vi "Write and Read Multiple Holding Registers.vi"(4 "read count":u16, 6 "read operation starting address":u16, 8 "error in (no error)":errorcluster, 9 "values to write":u16[](array[numeric]), 10 "write operation starting address":u16, 11 "Modbus master in":refnum<class "Network Master.lvclass">) -> (0 "error out":errorcluster, 1 "values read":u16[](array[numeric]), 3 "Modbus master out":refnum<class "Network Master.lvclass">)   [LabVIEW 2021, in "Network Master.lvclass"]
doc: "Writes and reads values to and from contiguous holding registers. This VI performs the write operation before the read operation. The maximum number of holding registers this VI can write is 121. The maximum number of holding registers this VI can read is 125."
uses:
  Network Master.lvclass
  D:/my_projects/projects/Algorithms/Labview/21/Modbus_v121c/Network Protocol/Network Protocol.lvclass
  Modbus Data Unit/Modbus Data Unit.lvclass/Modbus Data Unit.ctl
  Network Protocol.lvclass/Network Protocol.ctl
  Network Master.lvclass/Network Master.ctl
  Modbus Data Unit/Construct PDU.vi
  Utility/U16s to Bytes.vi
  Utility/Bytes to U16s.vi
  Master Function Definition/Function code mismatch error.vi
  Data Model/Error Generator.vi
  Modbus Data Unit/Deconstruct PDU.vi
  Read Transmission Data Unit.vi
  Modbus Data Unit/Modbus Data Unit.lvclass
  Transmission Data Unit/Transmission Data Unit.lvclass
  Master Function Definition/Master Function Definition.lvclass
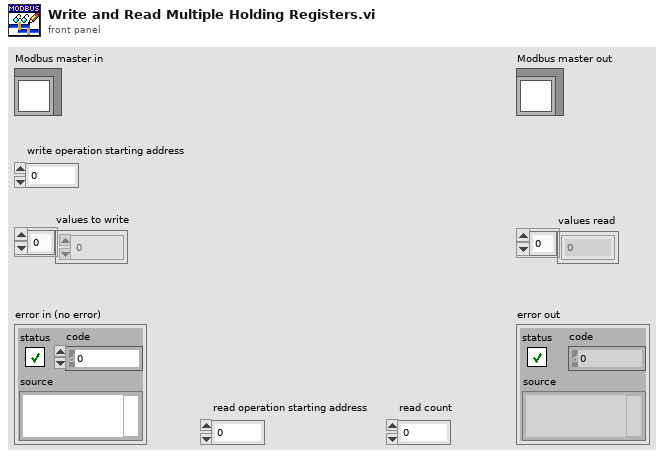
[diagram p1: front panel]
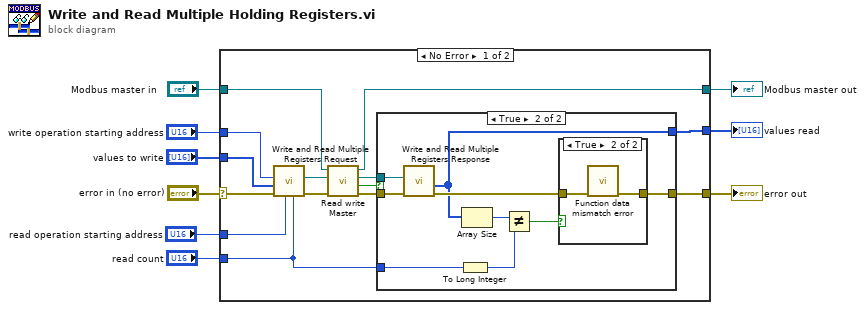
[diagram p0: block diagram]
diagram:
  n1 = case shown="No Error" "error in (no error)" {
    selector: "error in (no error)" -> [w12 w37]
    tunnel: "Modbus master in" -> [w10 w38]
    tunnel: [w11 w38] -> w8
    tunnel: [w22 w37] -> w7
    tunnel: "read count" -> [w20 _]
    tunnel: [w19 _] -> w4
    tunnel: "read operation starting address" -> [w18 _]
    tunnel: "values to write" -> [w17 _]
    tunnel: "write operation starting address" -> [w16 _]
    frame No Error {
      n2 = call "Write and Read Multiple Registers Request.vi"("Quantity to Read"=w20, "Read Starting Address"=w18, "error in"=w12, "Write"=w17, "Write Starting Address"=w16) -> ("error out"=w23:errorcluster, "modbus data unit out"=w13:refnum<class "Modbus Data Unit.lvclass">)  [unwired: 5 in]
      n3 = call "Read write Master.vi"("error in (no error)"=w23, "Modbus data unit in"=w13, "Modbus master in"=w10) -> ("error out"=w21:errorcluster, "PDU valid?"=w15:bool, "Modbus data unit out"=w14:refnum<class "Modbus Data Unit.lvclass">, "Modbus master out"=w11:refnum<class "Network Master.lvclass">)  [unwired: 5 in]
      n4 = case shown="True" w15 {
        tunnel: [w24 w33] -> w22
        tunnel: w21 -> [w24 w32]
        tunnel: w14 -> [_ w31]
        tunnel: w20 -> [_ w27]
        tunnel: [_ w26] -> w19
        frame False {
        }
        frame True {
          n5 = call "Write and Read Multiple Registers Response.vi"("error in"=w32, "modbus data unit in"=w31) -> ("error out"=w30:errorcluster, "Registers"=w26:u16[])  [unwired: 7 in, 1 out]
          n6 = To Long Integer(number=w27) -> (32bit integer=w25:i32)
          n7 = Array Size(array=w26) -> (size(s)=w28:i32)
          n8 = Not Equal?(x=w28, y=w25) -> (x != y?=w29:bool)
          n9 = case shown="True" w29 {
            tunnel: [w34 w36] -> w33
            tunnel: w30 -> [w34 w35]
            frame False {
            }
            frame True {
              n10 = call "Function data mismatch error.vi"("error in (no error)"=w35) -> ("error out"=w36:errorcluster)  [unwired: 10 in]
            }
          }
        }
      }
    }
    frame Error {
    }
  }
  "error out" <- w7
  "Modbus master out" <- w8
  "values read" <- w4
